vi "write frame data.vi"(8 "error in":errorcluster, 10 "frame data":T1, 11 "file string in":string) -> (0 "error out":errorcluster, 3 "file string out":string)   [LabVIEW 2018, in "Data Parser.lvclass"]
uses:
  Data Parser.lvclass
  frame data.ctl
  frame title.ctl
  frame basic data.ctl
  frame o data.ctl
  frame bp data.ctl
  frame c data.ctl
  frame w data.ctl
  frame i data.ctl
  frame b data.ctl
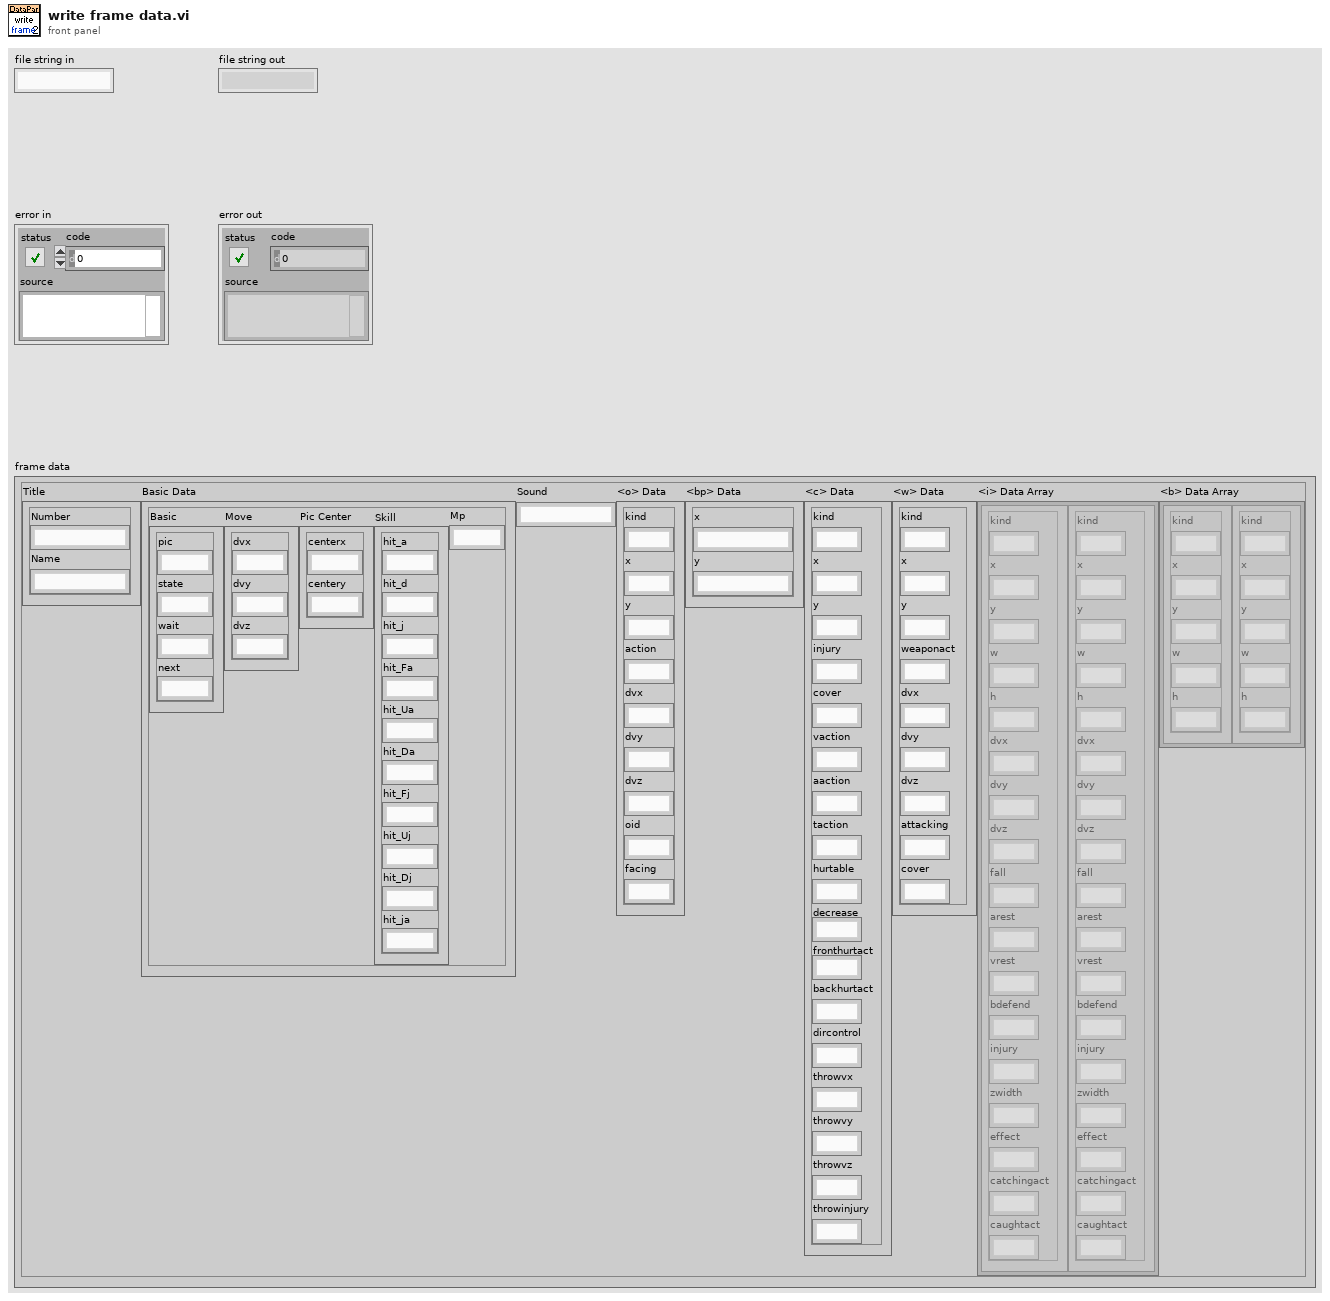
[diagram p1: front panel]
types:
  T1 = typedef "Data Parser.lvclass/frame data.ctl" = cluster{"Title":T2, "Basic Data":T3, "Sound":string, "<o> Data":T4, "<bp> Data":T5, "<c> Data":T6, "<w> Data":T7, "<i> Data Array":T8[], "<b> Data Array":T9[]}
  T2 = typedef "Data Parser.lvclass/frame title.ctl" = cluster{"Number":string, "Name":string}
  T3 = typedef "Data Parser.lvclass/frame basic data.ctl" = cluster{"Basic":cluster{"pic":string, "state":string, "wait":string, "next":string}, "Move":cluster{"dvx":string, "dvy":string, "dvz":string}, "Pic Center":cluster{"centerx":string, "centery":string}, "Skill":cluster{"hit_a":string, "hit_d":string, "hit_j":string, "hit_Fa":string, "hit_Ua":string, "hit_Da":string, "hit_Fj":string, "hit_Uj":string, "hit_Dj":string, "hit_ja":string}, "Mp":string}
  T4 = typedef "Data Parser.lvclass/frame o data.ctl" = cluster{"kind":string, "x":string, "y":string, "action":string, "dvx":string, "dvy":string, "dvz":string, "oid":string, "facing":string}
  T5 = typedef "Data Parser.lvclass/frame bp data.ctl" = cluster{"x":string, "y":string}
  T6 = typedef "Data Parser.lvclass/frame c data.ctl" = cluster{"kind":string, "x":string, "y":string, "injury":string, "cover":string, "vaction":string, "aaction":string, "taction":string, "hurtable":string, "decrease":string, "fronthurtact":string, "backhurtact":string, "dircontrol":string, "throwvx":string, "throwvy":string, "throwvz":string, "throwinjury":string}
  T7 = typedef "Data Parser.lvclass/frame w data.ctl" = cluster{"kind":string, "x":string, "y":string, "weaponact":string, "dvx":string, "dvy":string, "dvz":string, "attacking":string, "cover":string}
  T8 = typedef "Data Parser.lvclass/frame i data.ctl" = cluster{"kind":string, "x":string, "y":string, "w":string, "h":string, "dvx":string, "dvy":string, "dvz":string, "fall":string, "arest":string, "vrest":string, "bdefend":string, "injury":string, "zwidth":string, "effect":string, "catchingact":string, "caughtact":string}
  T9 = typedef "Data Parser.lvclass/frame b data.ctl" = cluster{"kind":string, "x":string, "y":string, "w":string, "h":string}
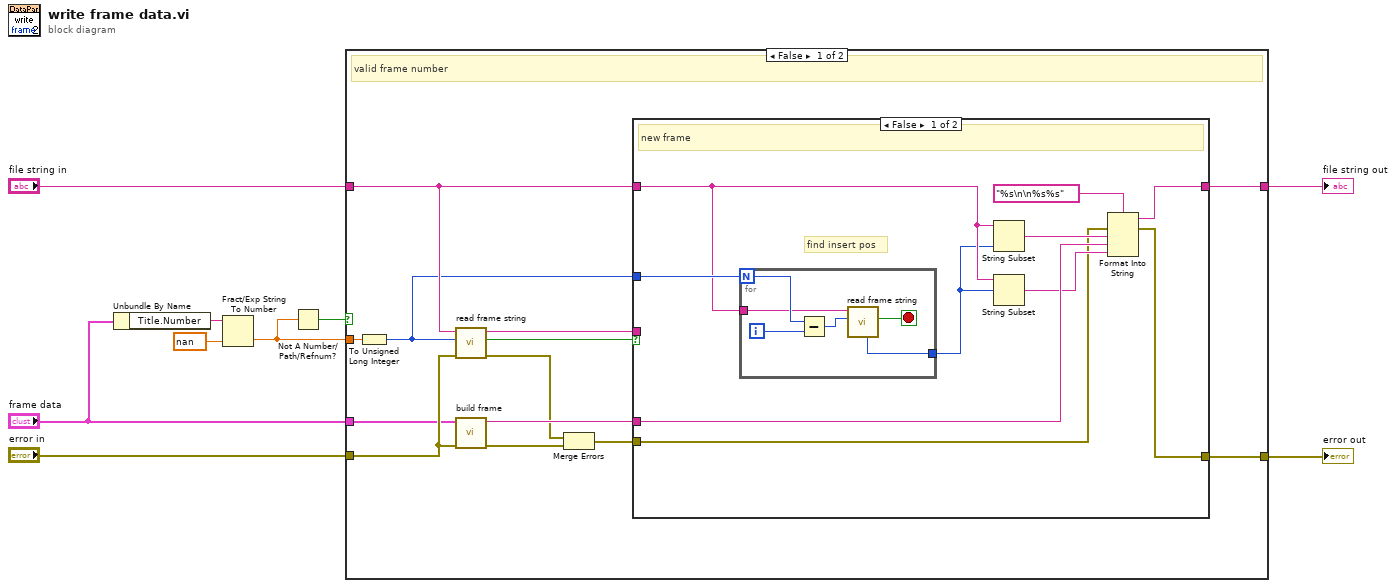
[diagram p0: block diagram]
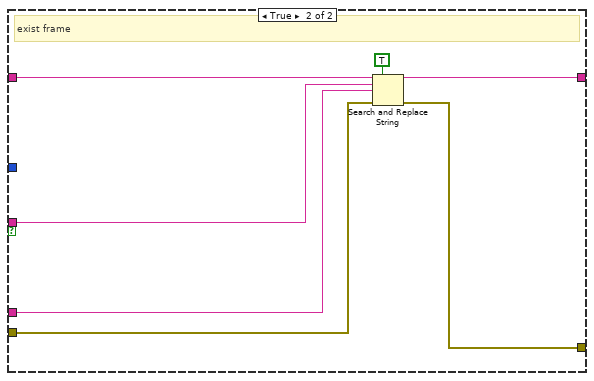
[diagram p2: hidden frame]
diagram:
  n1 = Unbundle By Name("frame data") -> ("Title.Number"=w3:string)
  n2 = Fract/Exp String To Number(string=w3, default (0 dbl)=nan) -> (number=w2:dbl)  [unwired: 2 in, 1 out]
  n3 = Not A Number/Path/Refnum?(number/path/refnum=w2) -> (NaN/Path/Refnum?=w1:bool)
  n4 = case shown="False" w1 {
    tunnel: "file string in" -> [w20 w46]
    tunnel: [w19 w46] -> w8
    tunnel: [w14 w47] -> w7
    tunnel: "error in" -> [w13 w47]
    tunnel: "frame data" -> [w12 _]
    tunnel: w2 -> [w11 _]
    frame False {
      # "valid frame number"
      n5 = To Unsigned Long Integer(number=w11) -> (unsigned 32bit integer=w10:u32)
      n6 = call "read frame string.vi"("error in"=w13, "frame number"=w10, "file string"=w20) -> ("error out"=w16:errorcluster, "found"=w18:bool, "<f> string"=w22:string)  [unwired: 5 in, 1 out]
      n7 = call "build frame.vi"("error in (no error)"=w13, "frame data"=w12) -> ("error out"=w17:errorcluster, "<f> string"=w21:string)  [unwired: 8 in]
      n8 = Merge Errors(w16, w17) -> (w15:errorcluster)
      n9 = case shown="False" w18 {
        tunnel: w22 -> [_ w45]
        tunnel: w21 -> [w27 w44]
        tunnel: w20 -> [w31 w42]
        tunnel: [w25 w41] -> w19
        tunnel: w10 -> [w32 _]
        tunnel: w15 -> [w24 w40]
        tunnel: [w23 w39] -> w14
        frame False {
          # "find insert pos"
          # "new frame"
          n10 = for {
            N: w32 -> [w38]
            tunnel: w31 -> [w35]
            tunnel: [w34] -> w30
            i -> [w37]
            stop <- w33 stop-if-true
            n11 = Subtract(x=w38, y=w37) -> (x-y=w36:i32)
            n12 = call "read frame string.vi"("frame number"=w36, "file string"=w35) -> ("found"=w33:bool, "<f> end pos"=w34:i32)  [unwired: 6 in, 2 out]
          }
          n13 = String Subset(string=w31, length (rest)=w30) -> (substring=w28:string)  [unwired: 1 in]
          n14 = String Subset(string=w31, offset (0)=w30) -> (substring=w26:string)  [unwired: 1 in]
          n15 = Format Into String(format string="%s\n\n%s%s", error in=w24, w28, w27, w26) -> (resulting string=w25:string, error out=w23:errorcluster)  [unwired: 1 in]
        }
        frame True {
          # "exist frame"
          n16 = Search and Replace String(replace all?=TRUE ("replace all? (F)"), input string=w42, search string=w45, replace string=w44, error in=w40) -> (result string=w41:string, error out=w39:errorcluster)  [unwired: 3 in, 2 out]
        }
      }
    }
    frame True {
      # "invalid frame number"
    }
  }
  "file string out" <- w8
  "error out" <- w7
